vi "Get Series Enqueuer.vi"(8 "error in":errorcluster, 11 "Study Actor in":refnum<class "Study Actor.lvclass">) -> (0 "error out":errorcluster, 2 "Enqueuer":refnum<class "Message Enqueuer.lvclass">, 3 "Study Actor out":refnum<class "Study Actor.lvclass">)   [LabVIEW 2024, in "Study Actor.lvlib" / "Study Actor.lvclass"]
uses:
  Study Actor.lvclass
  <vilib>/ActorFramework/Message Enqueuer/Message Enqueuer.lvclass
  Study Actor.lvclass/Study Actor.ctl
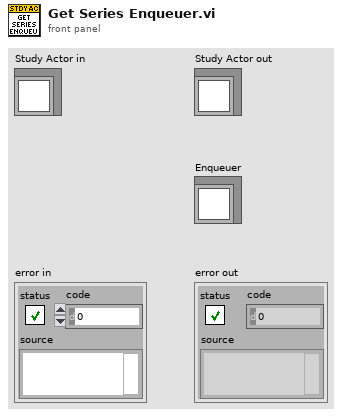
[diagram p1: front panel]
types:
  T1 = map{string, refnum<class "Message Enqueuer.lvclass">}
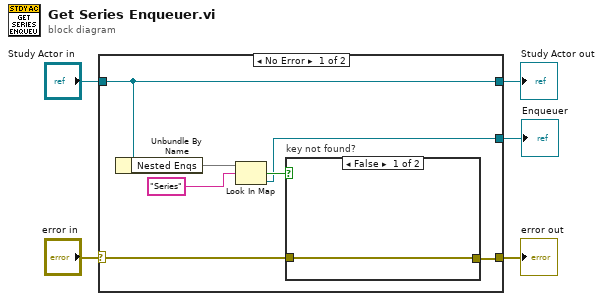
[diagram p0: block diagram]
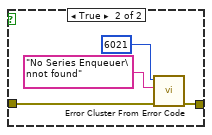
[diagram p2: hidden frame]
diagram:
  n1 = case shown="No Error" "error in" {
    selector: "error in" -> [w7 w19]
    tunnel: [w9 w19] -> w4
    tunnel: [w12 w18] -> w2
    tunnel: "Study Actor in" -> [w12 w18]
    tunnel: [w6 _] -> w1
    frame No Error {
      n2 = Unbundle By Name(w12) -> ("Nested Enqs"=w11:T1)
      n3 = Look In Map(map=w11, key="Series") -> (key not found?=w8:bool, value=w6:refnum<class "Message Enqueuer.lvclass">)  [unwired: 1 in]
      n4 = case "key not found?" shown="False" w8 {
        tunnel: [w13 w16] -> w9
        tunnel: w7 -> [w13 w17]
        frame False {
        }
        frame True {
          n5 = call <vilib>:"Error Cluster From Error Code.vi"("error in (no error)"=w17, "error message (\"\")"="No Series Enqueuer\nnot found" ("error message (\"\")"), "error code (0)"=6021) -> ("error out"=w16:errorcluster)  [unwired: 6 in]
        }
      }
    }
    frame Error {
    }
  }
  "error out" <- w4
  "Study Actor out" <- w2
  "Enqueuer" <- w1
